vi "test Set AccessType.vi"(11 "Test Case In":refnum<class "Test Object Entry.lvclass">) -> (0 "error out":errorcluster, 3 "Test Case Out":refnum<class "Test Object Entry.lvclass">)   [LabVIEW 2020, in "Test Object Entry.lvclass"]
uses:
  Test Object Entry.lvclass
  C:/Program Files/National Instruments/LabVIEW 2026/vi.lib/Astemes/LUnit/Test Case.lvclass
  source/Object Dictionary/Object Dictionary.lvclass
  source/Object Entry/Object Entry.lvclass/Object Entry.ctl
  source/Sub Object/Sub Object.lvclass/Sub Object.ctl
  <vilib>/Astemes/LUnit/Test Case.lvclass/Test Case.ctl
  source/Sub Objects Dictionary/Sub Objects Dictionary.lvclass
  source/Object Entry/Object Entry.lvclass
  source/Typedefs/Access Type.ctl
  source/CANopen.lvlib
  <vilib>/Astemes/LUnit/Test Case.lvclass
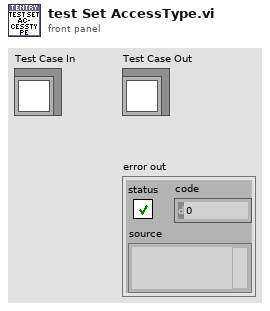
[diagram p1: front panel]
types:
  T1 = typedef "CANopen.lvlib/Access Type.ctl" = enum16{"unknown", "ro", "wo", "rw", "rwr", "rww", "const"}
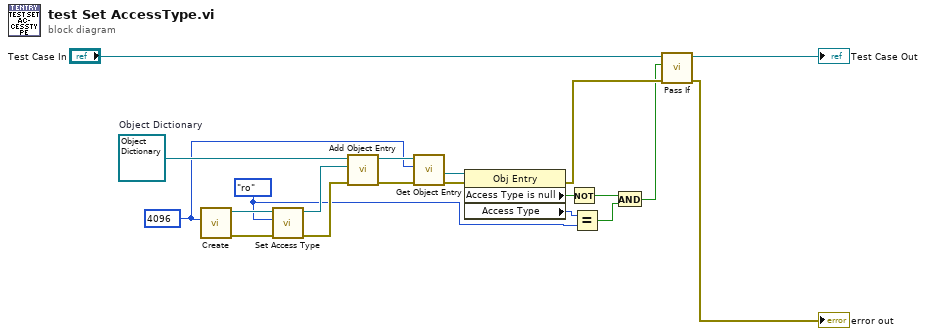
[diagram p0: block diagram]
diagram:
  w2 = Access_Type."ro" ("Access Type")
  w10 = u16 4096 ("Index")
  w17 = refnum<class "Object Dictionary.lvclass"> refnum  # Object Dictionary
  n1 = call "Create.vi"("Index"=w10) -> ("error out"=w16:errorcluster, "Object Entry"=w15:refnum<class "Object Entry.lvclass">)  [unwired: 9 in]
  n2 = call "Set Access Type.vi"("error in"=w16, "Access Type"=w2, "Object Entry in"=w15) -> ("error out"=w13:errorcluster, "Object Entry out"=w14:refnum<class "Object Entry.lvclass">)  [unwired: 7 in]
  n3 = call "Add Object Entry.vi"("error in"=w13, "Obj Entry"=w14, "Obj Dict in"=w17) -> ("error out"=w12:errorcluster, "Obj Dict out"=w11:refnum<class "Object Dictionary.lvclass">)  [unwired: 7 in]
  n4 = call "Get Object Entry.vi"("error in"=w12, "OD Index"=w10, "Obj Dict in"=w11) -> ("error out"=w9:errorcluster, "Obj Entry"=w8:refnum<class "Object Entry.lvclass">)  [unwired: 6 in, 1 out]
  n5 = property class="Obj Entry"(reference=w8, error in=w9) -> (error out=w6:errorcluster, "Access Type is null"=w7:bool, "Access Type"=w3:T1)  [unwired: 1 out]
  n6 = Not(x=w7) -> (.not. x?=w5:bool)
  n7 = Equal?(x=w3, y=w2) -> (x = y?=w4:bool)
  n8 = And(x=w5, y=w4) -> (x .and. y?=w1:bool)
  n9 = call <vilib>:"Pass If.vi"("error in (no error)"=w6, "Pass?"=w1, "LUnit Test Case In"="Test Case In") -> ("error out"=→"error out":errorcluster, "LUnit Test Case Out"=→"Test Case Out":refnum<class "Test Object Entry.lvclass">)  [unwired: 7 in]
